vi "Select Channel.vi"(8 "error in (no error)":errorcluster, 9 "Table Name":string, 10 "Select Channels":string[](array[string]), 11 "Data Load Interface in":refnum<class "Data Load Interface.lvclass">) -> (0 "error out":errorcluster, 3 "Data Load Interface out":refnum<class "Data Load Interface.lvclass">)   [LabVIEW 2020, in "Data Load Interface.lvclass"]
uses:
  Data Load Interface.lvclass
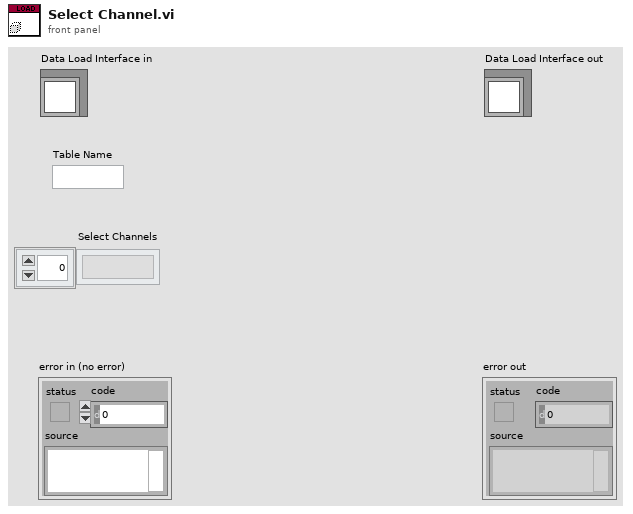
[diagram p1: front panel]
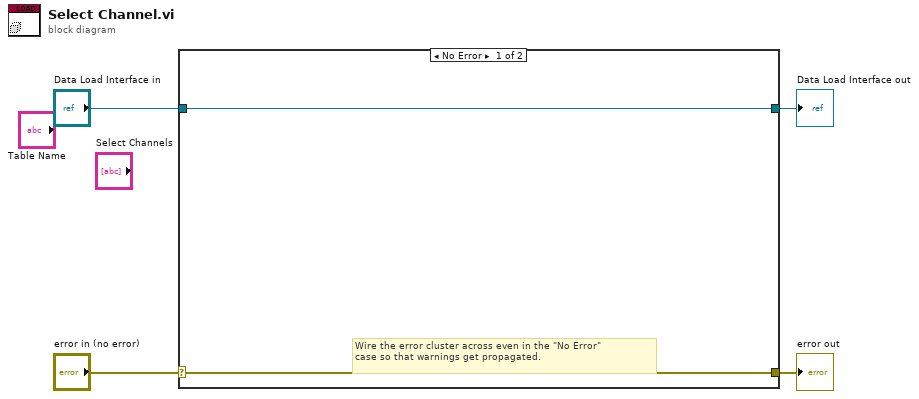
[diagram p0: block diagram]
diagram:
  n1 = case shown="No Error" "error in (no error)" {
    selector: "error in (no error)" -> [w5 w8]
    tunnel: [w5 w8] -> w3
    tunnel: [w6 w7] -> w1
    tunnel: "Data Load Interface in" -> [w6 w7]
    frame No Error {
      # "Wire the error cluster across even in the \"No Error\"\ncase so that warnings get propagated."
    }
    frame Error {
    }
  }
  "error out" <- w3
  "Data Load Interface out" <- w1
